vi "test9.vi"   [LabVIEW 2012]
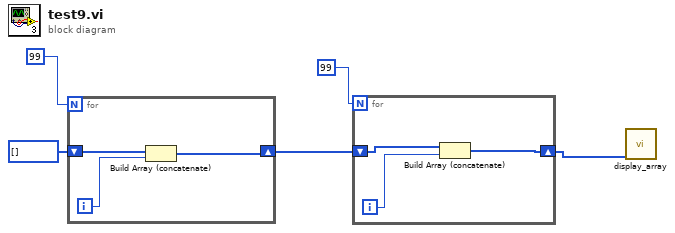
[diagram p0: block diagram]
diagram:
  n1 = for {
    N: 99 -> [_]
    shift-right: [w7] -> w5
    shift-left: i32[] [] -> [w8]
    i -> [w6]
    n2 = Build Array (concatenate)(w8, w6) -> (w7:i32[])
  }
  n3 = for {
    N: 99 -> [_]
    shift-right: [w10] -> w1
    shift-left: w5 -> [w11]
    i -> [w9]
    n4 = Build Array (concatenate)(w11, w9) -> (w10:i32[])
  }
  n5 = call "display_array.vi"("array"=w1) -> ()  [unwired: 10 in, 1 out]
